vi "DigLeCroyData.vi"(5 "Ring":u16(ring) items=["y-x scan", "x-y scan", "z-x scan", "y-z"], 6 "Total steps in line":i32, 7 "HP33120PRF ?":bool, 8 "Therapy (T)":bool, 9 "File Name In":string, 11 "Type of scan":u16(ring) items=["Therapy with scan", "M scan", "M scan w/ therapy", "1-D B Scan", "1-D B Scan w/ Therapy", "2-D B Scan", "2-D B Scan w/ Therapy"]) -> (0 "Error Message":string, 2 "Data":sgl[][][](array[numeric]), 3 "Scan Params":T1={"Header Version"="", "Header Length"=0, "rf points per line"=0, "lines per scan"=0, "Sampling Rate (MHz)"=0, "bits A/D"=0, "Bytes A/D"=0, "Digitizer"="", "File Name"="", "Att Array"=[], "date string"="", "time string"="", "Patient ID"="", "Number of Scans"=0, "avg num"=0.0, "Keep?"=FALSE, "Digitizer delay\n (ms) "=0.0, "Therapy Parameters"={"Theraputic Freq (MHz)"=1.0, "Time on"=0.0, "Therapy amplitude (mV)"=50.0, "Lines Before"=0, "Lines After"=0}, "Scan Settings"={"ENERGY(UJ)"=0, "DAMPING (IN Ohm)"=0, "HP FILT(IN KHz) "=0, "LP FILT(IN MHz)"=0, "GAIN(db)"=0, "prf (kHz)"=0.0, "Distance between\nscan lines (mm)"=0, "Distance between\nscan planes (mm)"=0}} {"Scan Settings"."prf (kHz)" format="%.2f"; "Scan Settings"."GAIN(db)" items=["26.0", "40.0", "54.0"]; "Scan Settings"."LP FILT(IN MHz)" items=["20", "50", "100", "200"]; "Scan Settings"."HP FILT(IN KHz)" items=["1", "1000", "3000", "10000"]; "Scan Settings"."DAMPING (IN Ohm)" items=["7", "10", "16", "20", "26", "30", "40", "50"]; "Scan Settings"."ENERGY(UJ)" items=["1", "2", "4", "8", "16", "32"]; "Therapy Parameters"."Therapy amplitude (mV)" format="%.2f"; "Therapy Parameters"."Time on" format="%.2f"; "Therapy Parameters"."Theraputic Freq (MHz)" format="%.2f"; "Digitizer delay\n (ms)" format="%.2f"; "avg num" format="%.2f"})   [LabVIEW 2022 SP3]
uses:
  Motion Controllers/-MotionRoutines/MotionGlobals.vi
  LCDSO Single/Stop.vi
panel:
  out "Data":i8[][][](array[numeric])
  out "Raw data":sgl[](graph)
  in  "VISA session":refnum<visa-resource-name>="GPIB::4"
  # "First axis used in 1-D\nscan"
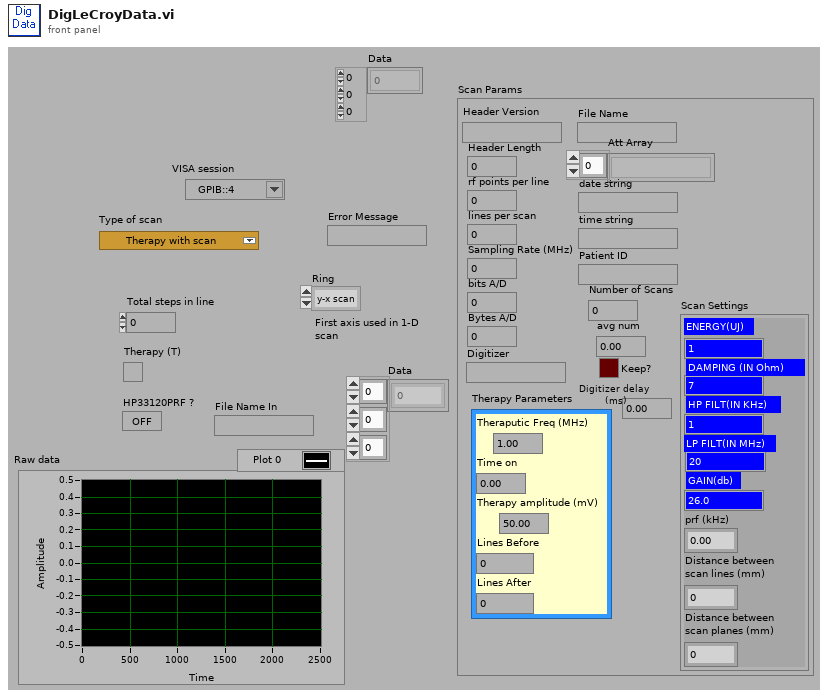
[diagram p1: front panel]
types:
  T1 = cluster{"Header Version":string, "Header Length":i32, "rf points per line":u16, "lines per scan":u16, "Sampling Rate (MHz)":i32, "bits A/D":i32, "Bytes A/D":i32, "Digitizer":string, "File Name":string, "Att Array":string[], "date string":string, "time string":string, "Patient ID":string, "Number of Scans":i32, "avg num":dbl, "Keep?":bool, "Digitizer delay\n (ms) ":dbl, "Therapy Parameters":cluster{"Theraputic Freq (MHz)":sgl, "Time on":sgl, "Therapy amplitude (mV)":sgl, "Lines Before":u16, "Lines After":u16}, "Scan Settings":cluster{"ENERGY(UJ)":u8, "DAMPING (IN Ohm)":u8, "HP FILT(IN KHz) ":u8, "LP FILT(IN MHz)":u8, "GAIN(db)":u8, "prf (kHz)":sgl, "Distance between\nscan lines (mm)":u16, "Distance between\nscan planes (mm)":u16}}
  T2 = enum16{"50", "100", "250", "500", "1000", "2500", "5K", "10K", "25K", "50K", "100K", "250K", "500K", "1M"}
  T3 = enum16{"500", "1000", "2500", "5000", "10k", "25k", "50k", "100K", "200K", "500K", "1M"}
  T4 = cluster{"SUBARRAY_COUNT":i32, "SWEEPS_PER_ACQ":i32, "POINTS_PER_PAIR":i16, "PAIR_OFFSET":i16, "VERTICAL_GAIN":sgl, "VERTICAL_OFFSET":sgl, "MAX_VALUE":sgl, "MIN_VALUE":sgl, "NOMINAL_BITS":i16, "NOM_SUBAR_CNT":i16}
  T5 = cluster{"TIMEBASE":i16, "VERT_COUPLING":i16, "PROBE_ATT":sgl, "FIXED_VERT_GAIN":i16, "BANDWIDTH_LIM":i16, "VERTICAL_VERN":sgl, "ACQ_VERT_OFFS":sgl, "WAVE_SOURCE":i16}
  T6 = cluster{"t(0) (sec)":ext, "Delta t (sec)":dbl, "Amplitude Array (Volts)":sgl[]}
  T7 = cluster{"rf points per line":u16, "lines per scan":u16, "Sampling Rate (MHz)":i32, "bits A/D":i32, "File Name":string, "Patient ID":string, "Number of Scans":i32, "avg num":dbl, "Keep?":bool, "Digitizer delay\n (ms) ":dbl}
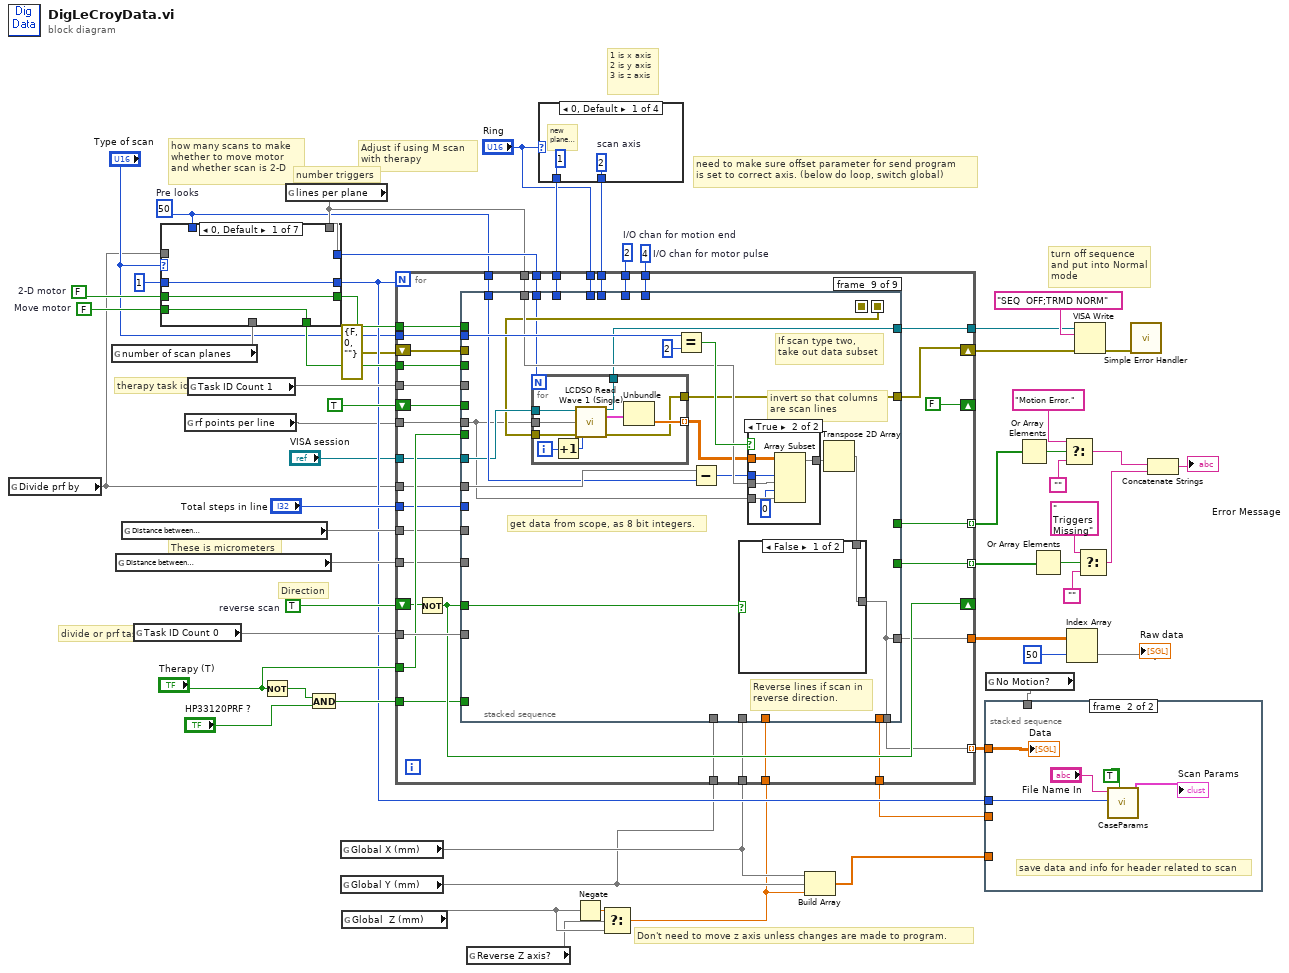
[diagram p0: block diagram]
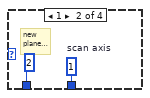
[diagram p2: hidden frame]
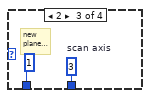
[diagram p3: hidden frame]
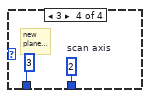
[diagram p4: hidden frame]
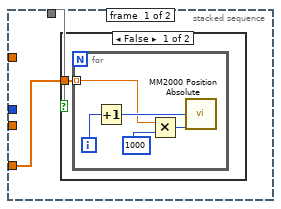
[diagram p5: hidden frame]
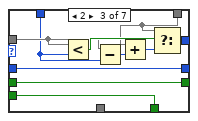
[diagram p8: hidden frame]
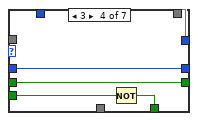
[diagram p9: hidden frame]
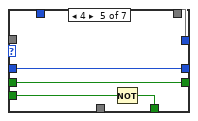
[diagram p10: hidden frame]
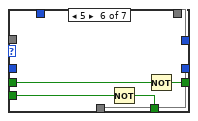
[diagram p11: hidden frame]
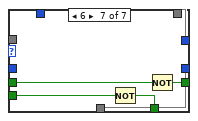
[diagram p12: hidden frame]
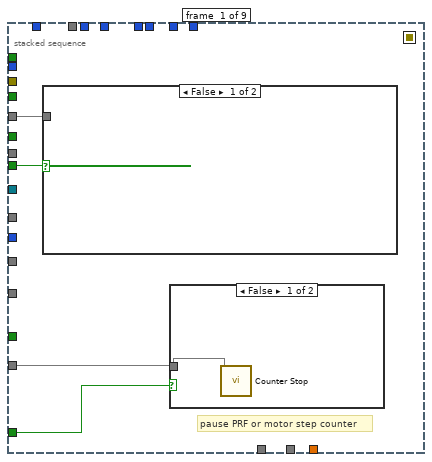
[diagram p13: hidden frame]
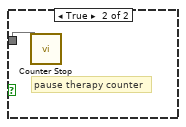
[diagram p15: hidden frame]
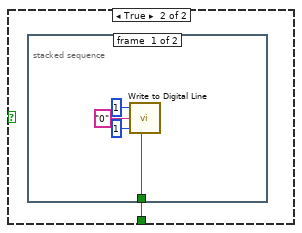
[diagram p17: hidden frame]
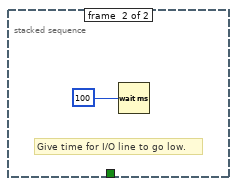
[diagram p18: hidden frame]
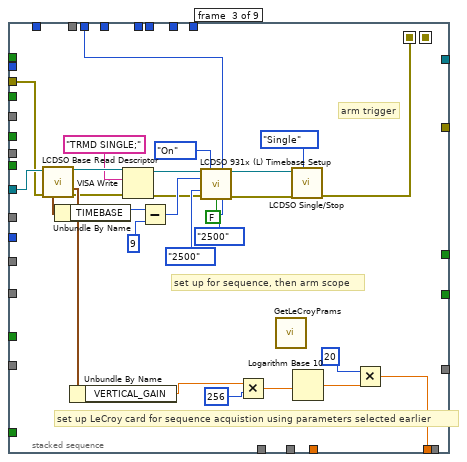
[diagram p19: hidden frame]
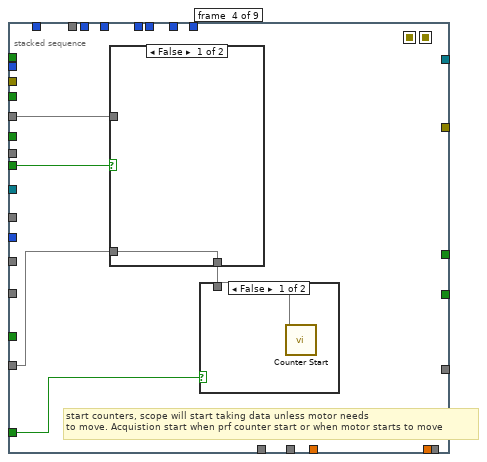
[diagram p20: hidden frame]
diagram:
  w24 = 50  # Pre looks
  w35 = 2  # I/O chan for motion end
  w34 = 4  # I/O chan for motor pulse
  w53 = TRUE  # reverse scan
  w55 = FALSE  # 2-D motor
  w56 = FALSE  # Move motor
  # "turn off sequence and put into Normal mode"
  # "1 is x axis\n2 is y axis\n3 is z axis"
  # "need to make sure offset parameter for send program\nis set to correct axis. (below do loop, switch global)"
  # "Adjust if using M scan\nwith therapy"
  # "Don't need to move z axis unless changes are made to program."
  # "These is micrometers"
  # "divide or prf task id"
  # "therapy task id"
  # "number triggers"
  # "Direction"
  # "how many scans to make\nwhether to move motor\nand whether scan is 2-D"
  n1 = global read "MotionGlobals.vi" "Divide prf by"() -> (w25)
  n2 = global read "MotionGlobals.vi" "number of scan planes"() -> (w58)
  n3 = global read "MotionGlobals.vi" "Distance between\nscan planes (mm)"() -> (w51)
  n4 = global read "MotionGlobals.vi" "Distance between\nscan lines (mm)"() -> (w52)
  n5 = global read "MotionGlobals.vi" "Task ID Count 0"() -> (w47)
  n6 = global read "MotionGlobals.vi" "rf points per line"() -> (w9)
  n7 = global read "MotionGlobals.vi" "Task ID Count 1"() -> (w48)
  n8 = Not(x="Therapy (T)") -> (.not. x?=w46:bool)
  n9 = global read "MotionGlobals.vi" "lines per plane"() -> (w26)
  n10 = case shown="0, Default" "Type of scan" {
    tunnel: [w63 w67 w77 w82 w87 w93 w99] -> w38
    tunnel: 1 -> [w63 w67 w77 w82 w87 _ _]
    tunnel: w58 -> [_ _ _ _ _ w93 w99]
    tunnel: [w62 w66 w76 w80 w85 w91 w97] -> w57
    tunnel: w56 -> [w62 w66 w76 w81 w86 w92 w98]
    tunnel: [w61 w65 w75 w79 w84 w89 w95] -> w54
    tunnel: w55 -> [w61 w65 w75 w79 w84 w90 w96]
    tunnel: [w60 w64 w73 w78 w83 w88 w94] -> w28
    tunnel: w26 -> [w60 w64 w70 w78 w83 w88 w94]
    tunnel: w25 -> [_ _ w69 _ _ _ _]
    tunnel: w24 -> [_ _ w68 _ _ _ _]
    frame 0, Default {
    }
    frame 1 {
    }
    frame 2 {
      n11 = Less?(x=w69, y=w68) -> (x < y?=w74:bool)
      n12 = Subtract(x=w69, y=w68) -> (x-y=w72:i32)
      n13 = Add(x=w70, y=w72) -> (x+y=w71:i32)
      n14 = Select(t=w70, s=w74, f=w71) -> (s? t:f=w73:i32)
    }
    frame 3 {
      n15 = Not(x=w81) -> (.not. x?=w80:bool)
    }
    frame 4 {
      n16 = Not(x=w86) -> (.not. x?=w85:bool)
    }
    frame 5 {
      n17 = Not(x=w92) -> (.not. x?=w91:bool)
      n18 = Not(x=w90) -> (.not. x?=w89:bool)
    }
    frame 6 {
      n19 = Not(x=w98) -> (.not. x?=w97:bool)
      n20 = Not(x=w96) -> (.not. x?=w95:bool)
    }
  }
  n21 = And(x=w46, y="HP33120PRF ?") -> (x .and. y?=w44:bool)
  n22 = global read "MotionGlobals.vi" "Global X (mm)"() -> (w23)
  n23 = global read "MotionGlobals.vi" "Global Y (mm)"() -> (w20)
  n24 = global read "MotionGlobals.vi" "Global  Z (mm)"() -> (w31)
  n25 = global read "MotionGlobals.vi" "Reverse Z axis?"() -> (w30)
  n26 = case shown="0, Default" "Ring" {
    tunnel: [1 ("Axis") 2 ("Axis") 1 ("Axis") 3 ("Axis")] -> w22
    tunnel: [w100 w102 w104 w106] -> w21
    frame 0, Default {
      w100 = 2  # scan axis
      # "new plane axis"
    }
    frame 1 {
      w102 = 1  # scan axis
      # "new plane axis"
    }
    frame 2 {
      w104 = 3  # scan axis
      # "new plane axis"
    }
    frame 3 {
      w106 = 2  # scan axis
      # "new plane axis"
    }
  }
  n27 = Negate(x=w31) -> (-x=w32:dbl)
  n28 = Select(t=w32, s=w30, f=w31) -> (s? t:f=w18:dbl)
  n29 = for {
    N: w38 -> [_]
    tunnel: w48 -> [w143]
    tunnel: w47 -> [w142]
    tunnel: "Therapy (T)" -> [w141]
    tunnel: w25 -> [w140]
    tunnel: w57 -> [w139]
    tunnel: w52 -> [w138]
    tunnel: w22 -> [w137]
    tunnel: w54 -> [w136]
    tunnel: w21 -> [w135]
    shift-right: [w133] -> _
    shift-left: w53 -> [w134]
    tunnel: w51 -> [w132]
    tunnel: w28 -> [w131]
    tunnel: w20 -> [w130]
    tunnel: "Total steps in line" -> [w129]
    tunnel: w35 -> [w128]
    tunnel: w23 -> [w127]
    shift-right: [FALSE] -> _
    shift-left: TRUE -> [w126]
    tunnel: w44 -> [w124]
    tunnel: w34 -> [w123]
    tunnel: [w122] -> w33 mode=indexing
    tunnel: w9 -> [w121]
    tunnel: [w120] -> w37 mode=indexing
    tunnel: [w119] -> w36
    tunnel: "Type of scan" -> [w118]
    tunnel: w26 -> [w117]
    tunnel: w24 -> [w116]
    tunnel: "Ring" -> [w115]
    tunnel: w18 -> [w114]
    tunnel: [w113] -> w14 mode=indexing
    shift-right: [w108] -> w6
    shift-left: errorcluster {"status"=FALSE, "code"=0, "source"=""} ("error out") -> [w112]
    tunnel: "VISA session" -> [w111]
    tunnel: [w110] -> w1
    tunnel: [w109] -> w4
    n30 = Not(x=w134) -> (.not. x?=w133:bool)
    n31 = stacked-sequence {
      seq-local: [_ _ w172 _ _ _ _ _ _] -> [_ _ _ _ _ w241 _ _ _]
      seq-local: [_ _ _ _ _ w241 _ _ _] -> [_ _ _ _ _ _ _ _ w272]
      tunnel: w141 -> [w145 _ _ w185 w207 _ w260 _ _]
      tunnel: w140 -> [_ _ _ _ _ _ _ _ w277]
      tunnel: w143 -> [w147 _ _ w189 _ _ w258 _ _]
      tunnel: w142 -> [w146 _ _ w188 _ _ w259 _ _]
      tunnel: w139 -> [_ w150 _ _ w211 _ _ w263 _]
      tunnel: w138 -> [_ _ _ _ w210 _ _ _ _]
      tunnel: w137 -> [_ _ _ _ w196 _ _ _ _]
      tunnel: w136 -> [_ _ _ _ w205 _ _ _ _]
      tunnel: w135 -> [_ _ _ _ w199 _ _ _ _]
      tunnel: w133 -> [_ w151 _ _ w209 _ _ _ w283]
      tunnel: w132 -> [_ _ _ _ w202 _ _ _ _]
      tunnel: w131 -> [_ _ w181 _ _ w239 _ _ w268]
      tunnel: w130 -> [_ _ _ _ w208 _ _ _ _]
      tunnel: w129 -> [_ _ _ _ w203 _ _ _ _]
      tunnel: w128 -> [_ _ _ _ w206 _ _ _ _]
      tunnel: w127 -> [_ _ _ _ w198 _ _ _ _]
      tunnel: w126 -> [_ _ _ _ w204 _ _ _ _]
      tunnel: w124 -> [w144 _ _ w186 _ _ w257 _ _]
      tunnel: w123 -> [_ _ _ _ w201 _ _ _ _]
      tunnel: [_ _ _ _ _ w242 _ _ _] -> w122
      tunnel: w121 -> [_ _ _ _ _ _ _ _ w269]
      tunnel: [_ _ _ _ _ _ _ _ w267] -> w120
      tunnel: [_ _ w158 _ _ _ _ _ _] -> w119
      tunnel: w118 -> [_ _ _ _ _ _ _ _ w280]
      tunnel: w117 -> [_ _ _ _ w200 _ _ _ w278]
      tunnel: w116 -> [_ _ _ _ _ _ _ _ w275]
      tunnel: w115 -> [_ _ _ _ w197 _ _ _ _]
      tunnel: w114 -> [_ _ _ _ w195 _ _ _ _]
      tunnel: [_ _ _ _ w194 _ _ _ _] -> w113
      tunnel: w112 -> [_ _ w168 _ _ _ _ _ _]
      tunnel: w111 -> [_ _ w179 _ _ w240 _ _ w273]
      tunnel: [_ _ _ _ _ _ _ _ w271] -> w110
      tunnel: [_ _ _ _ _ _ _ _ w267] -> w109
      tunnel: [_ _ _ _ _ _ _ _ w266] -> w108
      frame #0 {
        # "pause PRF or motor step counter"
        n32 = case shown="False" w145 {
          tunnel: w147 -> [_ w149]
          frame False {
          }
          frame True {
            # "pause therapy counter"
            n33 = call <vilib>:"Counter Stop.vi"("taskID"=w149) -> ()  [unwired: 5 in, 2 out]
          }
        }
        n34 = case shown="False" w144 {
          tunnel: w146 -> [w148 _]
          frame False {
            n35 = call <vilib>:"Counter Stop.vi"("taskID"=w148) -> ()  [unwired: 5 in, 2 out]
          }
          frame True {
          }
        }
      }
      frame #1 {
        # "Indicate if scan is in a reverse direction. For\nsome reason setting the I/O line high on the Nat Instr\nboard caused a trigger on the MM2K motor pulse line\nso this frame has to be executed before the DP100\nis armed to take data. Skip if not moving motors"
        n36 = case shown="False" w150 {
          tunnel: w151 -> [_ w152]
          frame False {
          }
          frame True {
            n37 = stacked-sequence {
              tunnel: w152 -> [w153 _]
              frame #0 {
                n38 = call <vilib>:"Write to Digital Line.vi"("device"=i16 1, "digital channel"="0", "line"=i16 1, "line state"=w153) -> ()  [unwired: 5 in]
              }
              frame #1 {
                # "Give time for I/O line to go low."
                n39 = Wait (ms)(milliseconds to wait=100) -> ()  [unwired: 1 out]
              }
            }
          }
        }
      }
      frame #2 {
        # "arm trigger"
        # "set up for sequence, then arm scope"
        # "set up LeCroy card for sequence acquistion using parameters selected earlier"
        n40 = call "LCDSO Base Read Descriptor.vi"("VISA session"=w179, "error in (no error)"=w168) -> ("dup VISA session"=w170:refnum<visa-resource-name>, "Parameters 3"=w174:T4, "Parameters 5"=w184:T5, "error out"=w167:errorcluster)  [unwired: 7 in, 3 out]
        n41 = Unbundle By Name(w184) -> ("TIMEBASE"=w183:i16)
        n42 = Unbundle By Name(w174) -> ("VERTICAL_GAIN"=w159:sgl)
        n43 = VISA Write(VISA resource name=w170, write buffer="TRMD SINGLE;", error in (no error)=w167) -> (VISA resource name out=w169:refnum<visa-resource-name>, error out=w166:errorcluster)  [unwired: 1 out]
        n44 = Subtract(x=w183, y=9) -> (x-y=w176:i32)
        n45 = call "LCDSO 931x (L) Timebase Setup.vi"("VISA session"=w169, "Sequence (0:Off)"=enum16{"Off", "On", "Wrap"}."On", "Segment count (2 samp.)"=w181, "Time/Div (17: 0.5 ms)"=w176, "Record Up To (0:500)"=T3."2500", "error in (no error)"=w166, "Sampling (F:Single Shot)"=FALSE, "Max.Seg.Size (1:100 samp.)"=T2."2500") -> ("dup VISA session"=w164:refnum<visa-resource-name>, "error out"=w173:errorcluster)  [unwired: 6 in]
        n46 = Multiply(x=w159, y=256) -> (x*y=w162:sgl)
        n47 = call "GetLeCroyPrams.vi"() -> ()  [unwired: 5 in, 7 out]
        n48 = call "LCDSO Single/Stop.vi"("Acquisition (0: Don't Care)"=enum16{"Don't Care", "Single", "Stop"}."Single", "error in (no error)"=w173, "VISA session"=w164) -> ("error out"=w172:errorcluster)  [unwired: 7 in, 1 out]
        n49 = Logarithm Base 10(1:w162) -> (0:w161:sgl)
        n50 = Multiply(x=20, y=w161) -> (x*y=w158:sgl)
      }
      frame #3 {
        # "start counters, scope will start taking data unless motor needs\nto move. Acquistion start when prf counter start or when motor starts to move"
        n51 = case shown="False" w185 {
          tunnel: w189 -> [_ w192]
          tunnel: w188 -> [w191 w193]
          tunnel: [w191 w193] -> w187
          frame False {
          }
          frame True {
            n52 = call <vilib>:"Counter Start.vi"("taskID"=w192) -> ()  [unwired: 9 in, 2 out]
          }
        }
        n53 = case shown="False" w186 {
          tunnel: w187 -> [w190 _]
          frame False {
            n54 = call <vilib>:"Counter Start.vi"("taskID"=w190) -> ()  [unwired: 9 in, 2 out]
          }
          frame True {
          }
        }
      }
      frame #4 {
        # "move motor if needed or move on"
        n55 = case shown="True" w211 {
          tunnel: w210 -> [_ w231]
          tunnel: w209 -> [_ w234]
          tunnel: w208 -> [_ w223]
          tunnel: w207 -> [_ w232]
          tunnel: w206 -> [_ w233]
          tunnel: w205 -> [_ w230]
          tunnel: w204 -> [_ w229]
          tunnel: w203 -> [_ w228]
          tunnel: w202 -> [_ w227]
          tunnel: w201 -> [_ w226]
          tunnel: w200 -> [_ w225]
          tunnel: w199 -> [_ w224]
          tunnel: w198 -> [_ w222]
          tunnel: w197 -> [_ w218]
          tunnel: w196 -> [_ w217]
          tunnel: w195 -> [_ w216]
          tunnel: [FALSE w215] -> w194
          frame False {
            # "use function generator prf"
            n56 = call <vilib>:"Write to Digital Line.vi"("line"=2, "line state"=FALSE) -> ()  [unwired: 7 in]
          }
          frame True {
            # "offset"
            # "assemble,send and execute\nmotion program. Some steps are\nskipped with 2-D motion. Compilation only occurs on first pass through index loop"
            # "move motor down axis"
            n57 = case shown="1" w218 {
              tunnel: w223 -> [w235 _ _ w238]
              tunnel: [w235 w236 w237 w238] -> w220
              tunnel: w222 -> [_ w236 _ _]
              tunnel: w216 -> [_ _ w237 _]
              frame 0, Default {
              }
              frame 1 {
              }
              frame 2 {
              }
              frame 3 {
              }
            }
            n58 = Multiply(x=1000, y=w220) -> (x*y=w219:i32)
            n59 = call "SendProgram.vi"("Type of scan"=w233, "Line Axis"=w224, "Avg Num"=w217, "lines per scan plane"=w225, "Reverse ?"=w234, "Therapy/AVG ?"=w232, 7:w228, 8:w227, "I/O chan for motor pulse"=w226, 12:w230, 13:w231, 14:w229, "Offset"=w219) -> ("Error Status"=w215:bool)  [unwired: 6 in]
          }
        }
      }
      frame #5 {
        # "Check to see if data acquistion is finished. Wait ten seconds\nmore and then exit if still no trigger. Data should all be taken be \nthe time this frame is reached. Stop acquisition if data not taken within 10 seconds."
        n60 = Tick Count (ms)() -> (millisecond timer value=w243:u32)
        n61 = while {
          tunnel: w243 -> [w253]
          tunnel: [w250] -> w242
          tunnel: w240 -> [w248]
          tunnel: w239 -> [w245]
          stop <- w252 stop-if-true
          n62 = Tick Count (ms)() -> (millisecond timer value=w256:u32)
          n63 = call "LCDSO Base Read Descriptor.vi"("VISA session"=w248) -> ("Parameters 3"=w247:T4)  [unwired: 8 in, 6 out]
          n64 = Subtract(x=w256, y=w253) -> (x-y=w255:u32)
          n65 = Unbundle By Name(w247) -> ("SUBARRAY_COUNT"=w244:i32)
          n66 = Less?(x=w255, y=10000) -> (x < y?=w251:bool)
          n67 = Equal?(x=w244, y=w245) -> (x = y?=w246:bool)
          n68 = Not(x=w251) -> (.not. x?=w250:bool)
          n69 = Compound Arithmetic op=OR(w246, w250) -> (w252:bool)
          n70 = Wait (ms)(milliseconds to wait=10) -> ()  [unwired: 1 out]
        }
      }
      frame #6 {
        # "stop counters again"
        n71 = case shown="False" w260 {
          tunnel: w258 -> [_ w262]
          frame False {
          }
          frame True {
            # "stop therapy counter"
            n72 = call <vilib>:"Counter Stop.vi"("taskID"=w262) -> ()  [unwired: 5 in, 2 out]
          }
        }
        n73 = case shown="False" w257 {
          tunnel: w259 -> [w261 _]
          frame False {
            n74 = call <vilib>:"Counter Stop.vi"("taskID"=w261) -> ()  [unwired: 5 in, 2 out]
          }
          frame True {
          }
        }
      }
      frame #7 {
        # "turn off function generator prf"
        n75 = case shown="False" w263 {
          frame False {
            n76 = call <vilib>:"Write to Digital Line.vi"("line"=2, "line state"=TRUE) -> ()  [unwired: 7 in]
          }
          frame True {
          }
        }
      }
      frame #8 {
        # "If scan type two,\ntake out data subset"
        # "Reverse lines if scan in \nreverse direction."
        # "invert so that columns\nare scan lines"
        # "get data from scope, as 8 bit integers."
        n77 = for {
          N: w268 -> [_]
          tunnel: [w285] -> w266
          tunnel: w273 -> [w292]
          tunnel: w272 -> [w291]
          tunnel: [w290] -> w271
          tunnel: w269 -> [w289]
          tunnel: [w287] -> w270 mode=indexing
          i -> [w286]
          n78 = Increment(x=w286) -> (x+1=w284:i32)
          n79 = call "LCDSO Read Wave 1 (Single).vi"("VISA session"=w292, "# Of Points (0)"=w289, "error in (no error)"=w291, "# Of Segments (0)"=w284) -> ("dup VISA session"=w290:refnum<visa-resource-name>, "Wave Output"=w288:T6, "error out"=w285:errorcluster)  [unwired: 6 in, 3 out]
          n80 = Unbundle(w288) -> ("Amplitude Array (Volts)"=w287:sgl[])  [unwired: 2 out]
        }
        n81 = Equal?(x=w280, y=2) -> (x = y?=w279:bool)
        n82 = Subtract(x=w277, y=w275) -> (x-y=w276:i32)
        n83 = case shown="True" w279 {
          tunnel: w270 -> [w293 w299]
          tunnel: [w293 w298] -> w282
          tunnel: w278 -> [_ w297]
          tunnel: w269 -> [_ w296]
          tunnel: w276 -> [_ w294]
          frame False {
          }
          frame True {
            n84 = Array Subset(array=w299, index (row)=w294, length (row)=w297, index (col)=0, length (col)=w296) -> (w298:sgl[][])
          }
        }
        n85 = Transpose 2D Array(2D array=w282) -> (transposed array=w274:sgl[][])
        n86 = case shown="False" w283 {
          tunnel: w274 -> [w300 w301]
          tunnel: [w300 w302] -> w267
          frame False {
          }
          frame True {
            n87 = for {
              tunnel: w301 -> [w304] mode=indexing
              tunnel: [w303] -> w302 mode=indexing
              n88 = Reverse 1D Array(array=w304) -> (reversed array=w303:sgl[])
            }
          }
        }
      }
    }
  }
  n89 = Build Array(w23, w20, w18) -> (w39:dbl[])
  n90 = global read "MotionGlobals.vi" "No Motion?"() -> (w29)
  n91 = stacked-sequence {
    tunnel: w39 -> [w306 _]
    tunnel: w38 -> [_ w317]
    tunnel: w37 -> [_ w313]
    tunnel: w36 -> [_ _]
    tunnel: w29 -> [w305 _]
    frame #0 {
      n92 = case shown="False" w305 {
        tunnel: w306 -> [w307 _]
        frame False {
          n93 = for {
            tunnel: w307 -> [w308] mode=indexing
            i -> [w311]
            n94 = Increment(x=w311) -> (x+1=w312:i32)
            n95 = Multiply(x=w308, y=1000) -> (x*y=w310:i32)
            n96 = call "MM2000 Position Absolute.vi"("Position Absolute"=w310, "Axis"=w312) -> ()  [unwired: 1 in]
          }
        }
        frame True {
        }
      }
    }
    frame #1 {
      # "save data and info for header related to scan"
      n97 = call "CaseParams.vi"(7:TRUE, "Number of Scans"=w317, "File Name In"="File Name In") -> ("Scan Params"=→"Scan Params":T7)  [unwired: 8 in]
      "Data" <- w313
    }
  }
  n98 = Or Array Elements(Boolean array=w14) -> (logical OR=w17:bool)
  n99 = Or Array Elements(Boolean array=w33) -> (logical OR=w42:bool)
  n100 = Select(t="Motion Error.", s=w17, f="") -> (s? t:f=w11:string)
  n101 = Index Array(array=w4, index (col)=50) -> (element=→"Raw data":sgl[])  [unwired: 1 in]
  n102 = VISA Write(VISA resource name=w1, write buffer="SEQ  OFF;TRMD NORM", error in (no error)=w6) -> (error out=w5:errorcluster)  [unwired: 2 out]
  n103 = Select(t=" Triggers Missing", s=w42, f="") -> (s? t:f=w13:string)
  n104 = call <vilib>:"Simple Error Handler.vi"("error in (no error)"=w5) -> ()  [unwired: 4 in, 5 out]
  n105 = Concatenate Strings(w11, w13) -> (→"Error Message":string)
